vi "AlliGator Add Multiple Source Image ROIs.vi"(7 "Header message":string, 8 "Error In":errorcluster, 9 "ROIs":T1[](array[typedef]) {"Contours"."Type" items=["No Selection", "Point", "Line", "Rectangle", "Oval", "Polygon", "Freehand Region", "Annulus", "Unused2", "Unused3", "Broken Line", "Freehand Line", "Rotated Rectangle"]}, 11 "ROI Mask Image Path":path) -> (0 "Error Out":errorcluster, 2 "Message":string)   [LabVIEW 2021, in "AlliGator ROIs.lvlib"]
doc: "Adds multiple Source Image ROIs to ROI storage."
uses:
  AlliGator ROIs.lvlib
  AlliGator ROI Manager Actions.ctl
  AlliGator Source Image ROI Storage [MULT] v3.vi
  Strings/Strings.lvlib
panel:
  # "see the AlliGator License on the block diagram (Ctrl+E or Window:Show Block Diagram)"
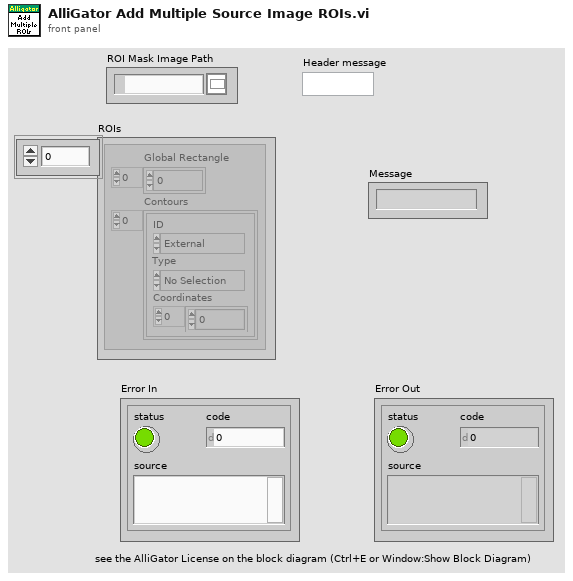
[diagram p1: front panel]
types:
  T1 = typedef "ROI Descriptor" = cluster{"Global Rectangle":i32[], "Contours":cluster{"ID":enum32{"External", "Internal"}, "Type":u32, "Coordinates":i32[]}[]}
  T2 = typedef "AlliGator ROIs.lvlib/AlliGator ROI Manager Actions.ctl" = enum16{"Undefined", "Delete Current ROI", "Delete All Unselected ROIs", "Delete Multiple ROIs", "Delete All ROIs", "Swap ROIs", "Insert ROI", "Update Current ROI Descriptor", "Rename Current ROI", "Store New ROI", "Store Multiple ROIs", "Select Next ROI", "Select Previous ROI", "Find Selected ROI", "Show All ROIs", "Update ROI Manager Window", "Merge All ROIs", "Unmerge ROI", "Set Selected ROI by ID"}
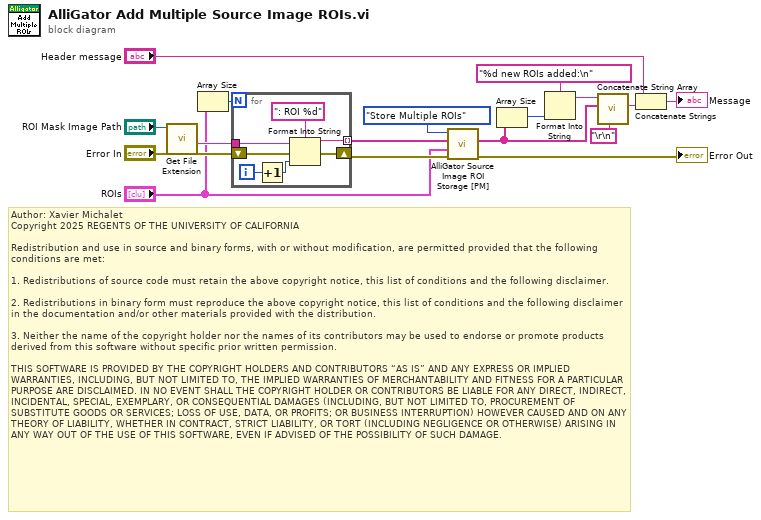
[diagram p0: block diagram]
diagram:
  # "Author: Xavier Michalet\nCopyright 2025 REGENTS OF THE UNIVERSITY OF CALIFORNIA\n\nRedistribution and use in source and binary forms, with or without modification, are permitted provided that the following conditions are met:\n\n1. Redistributions of source code must retain the above copyright notice, this list of conditions and the following disclaimer.\n\n2. Redistributions in binary form must reproduce the above copyright notice, this list of conditions and the following disclaimer in the documentation and/or other materials provided with the distribution.\n\n3. Neither the name of the copyright holder nor the names of its contributors may be used to endorse or promote products derived from this software without specific prior written permission.\n\nTHIS SOFTWARE IS PROVIDED BY THE COPYRIGHT HOLDERS AND CONTRIBUTORS “AS IS” AND ANY EXPRESS OR IMPLIED WARRANTIES, INCLUDING, BUT NOT LIMITED TO, THE IMPLIED WARRANTIES OF MERCHANTABILITY AND FITNESS FOR A PARTICULAR PURPOSE ARE DISCLAIMED. IN NO EVENT SHALL THE COPYRIGHT HOLDER OR CONTRIBUTORS BE LIABLE FOR ANY DIRECT, INDIRECT, INCIDENTAL, SPECIAL, EXEMPLARY, OR CONSEQUENTIAL DAMAGES (INCLUDING, BUT NOT LIMITED TO, PROCUREMENT OF SUBSTITUTE GOODS OR SERVICES; LOSS OF USE, DATA, OR PROFITS; OR BUSINESS INTERRUPTION) HOWEVER CAUSED AND ON ANY THEORY OF LIABILITY, WHETHER IN CONTRACT, STRICT LIABILITY, OR TORT (INCLUDING NEGLIGENCE OR OTHERWISE) ARISING IN ANY WAY OUT OF THE USE OF THIS SOFTWARE, EVEN IF ADVISED OF THE POSSIBILITY OF SUCH DAMAGE."
  n1 = call <vilib>:"Get File Extension.vi"("error in (no error)"="Error In", "file"="ROI Mask Image Path") -> ("error out"=w11:errorcluster, "filename without extension"=w10:string)  [unwired: 5 in, 3 out]
  n2 = Array Size(array="ROIs") -> (size(s)=w6:i32)
  n3 = for {
    N: w6 -> [_]
    tunnel: w10 -> [w25]
    shift-right: [w20] -> w9
    shift-left: w11 -> [w21]
    tunnel: [w19] -> w8 mode=indexing
    i -> [w23]
    n4 = Increment(x=w23) -> (x+1=w22:i32)
    n5 = Format Into String(format string=": ROI %d", initial string=w25, error in=w21, w22) -> (resulting string=w19:string, error out=w20:errorcluster)
  }
  n6 = call-poly "AlliGator Source Image ROI Storage [PM].vi"("Error In"=w9, "Current ROI Descriptors"="ROIs", "Default Names (\"ROI\")"=w8, "Action"=AlliGator_ROI_Manager_Actions."Store Multiple ROIs") -> ("Error Out"=→"Error Out":errorcluster, "Current ROI Names"=w15:string[])  [unwired: 2 in, 4 out]
  n7 = Array Size(array=w15) -> (size(s)=w13:i32)
  n8 = Format Into String(format string="%d new ROIs added:\n" ("Prefix (\"\")"), w13) -> (resulting string=w14:string)  [unwired: 2 in, 1 out]
  n9 = call "Concatenate String Array.vi"("Separator (TAB)"="\r\n", "String Array"=w15, "Prefix (\"\")"=w14) -> ("Formatted String"=w4:string)  [unwired: 8 in]
  n10 = Concatenate Strings("Header message", w4) -> (→"Message":string)
